vi "myRioStandarize.vi"(11 "Data in":dbl[](array[numeric])) -> (3 "Data out":dbl[](array[numeric]))   [LabVIEW 2019]
uses:
  Communication/TypeDef/#TypeDef_gForm.ctl
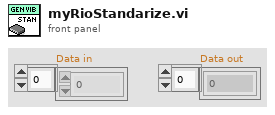
[diagram p1: front panel]
types:
  T1 = typedef "#TypeDef_gForm.ctl" = enum16{"1.5g", "6g"}
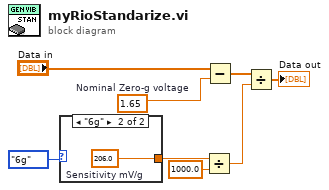
[diagram p0: block diagram]
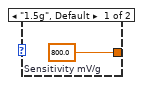
[diagram p2: hidden frame]
diagram:
  w4 = 1.65  # Nominal Zero-g voltage
  n1 = case shown="\"6g\"" #TypeDef_gForm."6g" {
    tunnel: [w9 w10] -> w6
    frame "1.5g", Default {
      w9 = 800.0  # Sensitivity mV/g
    }
    frame "6g" {
      w10 = 206.0  # Sensitivity mV/g
    }
  }
  n2 = Divide(x=w6, y=1000.0) -> (x/y=w1:dbl)
  n3 = Subtract(x="Data in", y=w4) -> (x-y=w2:dbl[])
  n4 = Divide(x=w2, y=w1) -> (x/y=→"Data out":dbl[])
